vi "VIs polimorficos.vi"() -> ()   [LabVIEW 2020]
panel:
  out "Suma de dos arreglos":i32[](array[numeric])
  out "Salida":i32[](array[numeric])
  out "Valor del Index":i32
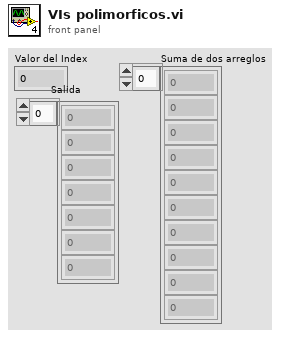
[diagram p1: front panel]
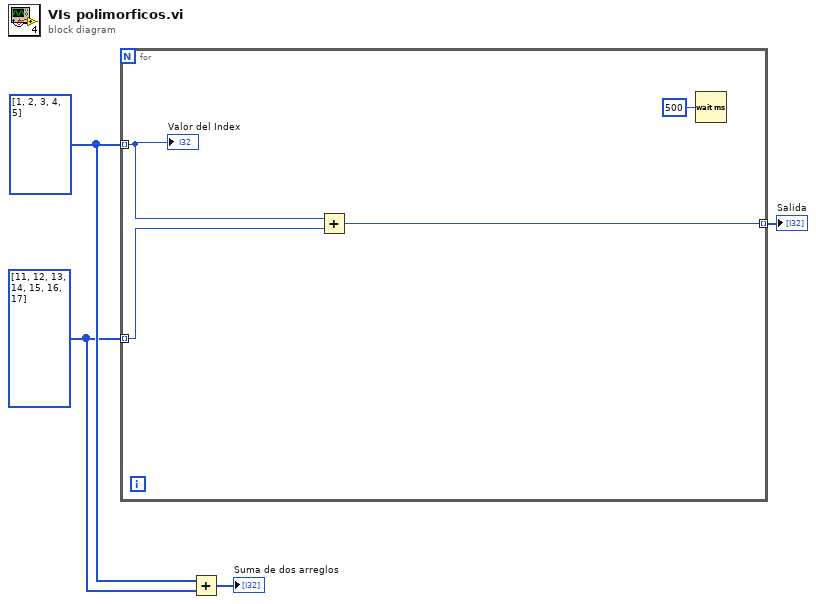
[diagram p0: block diagram]
diagram:
  w2 = i32[] [11, 12, 13, 14, 15, 16, 17]
  w3 = i32[] [1, 2, 3, 4, 5]
  n1 = for {
    tunnel: w3 -> [w6] mode=indexing
    tunnel: w2 -> [w7] mode=indexing
    tunnel: [w5] -> w4 mode=indexing
    n2 = Add(x=w6, y=w7) -> (x+y=w5:i32)
    n3 = Wait (ms)(milliseconds to wait=u32 500) -> ()  [unwired: 1 out]
    "Valor del Index" <- w6
  }
  "Salida" <- w4
  n4 = Add(x=w3, y=w2) -> (x+y=→"Suma de dos arreglos":i32[])
